vi "Get Params.vi"(8 "error in (no error)":errorcluster, 10 "Log Class":refnum<class "Build_Javier_Lopez_lib_Configuration_Filejson class.lvclass">, 11 "Module Meta in":refnum<class "Version.lvclass">) -> (0 "error out":errorcluster, 3 "Module Meta out":refnum<class "Version.lvclass">)   [LabVIEW 2021, in "Version.lvclass"]
uses:
  Version.lvclass
  <vilib>/Javier Lopez/Configuration File/Json Element/Build_Javier_Lopez_lib_Configuration_Filejson class.lvclass
  Version.lvclass/Version.ctl
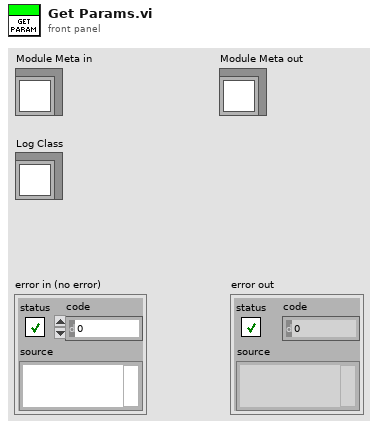
[diagram p1: front panel]
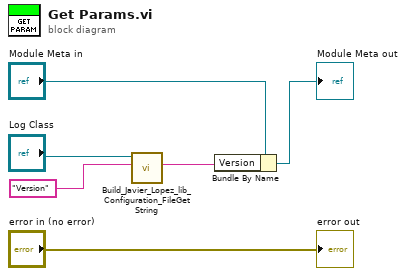
[diagram p0: block diagram]
diagram:
  n1 = call <vilib>:"Build_Javier_Lopez_lib_Configuration_FileGet String.vi"("Name"="Version", "json class in"="Log Class") -> ("String"=w1:string)  [unwired: 7 in, 2 out]
  n2 = Bundle By Name(cluster="Module Meta in", "Version"=w1) -> (→"Module Meta out":refnum<class "Version.lvclass">)
  "error out" <- "error in (no error)"
